vi "Oxford-IPS120-Main.vi"() -> ()   [LabVIEW 2016]
uses:
  IPS120 - SubVIs/Typedefs/Read System 1 - Enum.ctl
  IPS120 - SubVIs/Typedefs/Read System 2 - Enum.ctl
  IPS120 - SubVIs/Typedefs/Read Activity - Enum.ctl
  IPS120 - SubVIs/Typedefs/Read Switch Heater - Enum.ctl
  IPS120 - SubVIs/Typedefs/Read Mode 1 - Enum.ctl
  IPS120 - SubVIs/Typedefs/Read Mode 2 - Enum.ctl
  IPS120 - SubVIs/Typedefs/Set Control - Enum.ctl
  IPS120 - SubVIs/Typedefs/Set Switch Heater - Enum.ctl
  IPS120 - SubVIs/Typedefs/Set Activity - Enum.ctl
  <userlib>/_OpenG.lib/error/error.llb/Filter Error Codes (Array)__ogtk.vi
  API/IPS-120-API.lvlib
  IPS120 - SubVIs/IPS-120.lvlib
panel:
  in  "Tab Control":enum32{"Front Panel", "Error Log"}(tab)=enum."Error Log"
  out "input cluster":T7={"System 1"=enum."Normal", "System 2"=enum."Outside Positive Current Limi", "Activity"=enum."Hold", "Switch Heater"=enum."No Switch Fitted", "Mode 1"=enum."Amps Fast", "Mode 2"=enum."At Rest"}
  out "Magnet Current (A)":dbl=0.0006 format="%.4f"
  out "Voltage (V)":dbl(knob)=-0.0003 scale=-10.0..10.0
  out "Sentinel":bool=TRUE
  in  "Remote Mode":bool
  out "Power Supply Field (T)":dbl=0.0001 format="%#.5f"
  out "Magnet Field (T)":dbl format="%.5f"
  out "Voltage (V)":dbl=-0.0003 format="%.5f"
  out "PS Current (A)":dbl=0.0006 format="%.4f"
  in  "OK":bool
  out "Magnet Field (T)":dbl(knob) caption="Voltage (V)" scale=-20.0..20.0
  out "Switch Time":string="11:11:48"
  in  "PS Heat":bool
  in  "Clamp":bool
  in  "To Set":bool
  in  "To Zero":bool
  in  "Hold":bool
  out "Magnet Status":string="Clamped"
  out "Target Field Rate (T/min)":dbl=1.0 format="%.5f"
  out "Target Field (T)":dbl format="%#.5f"
  in  "Target Rate (T/min)":dbl=0.1 format="%.5f"
  in  "Target Field (T)":dbl format="%#.5f"
  in  "Send to IPS":bool
  out "Current (A)":dbl(knob)=0.0006 scale=-180.0..180.0
  out "Error List":T8(array[cluster])
  in  "IPS120 Address":refnum<visa-resource-name>="GPIB1::24::INSTR"
  # "Current (A)"
  # "Voltage (V)"
  # "Magnet (T)"
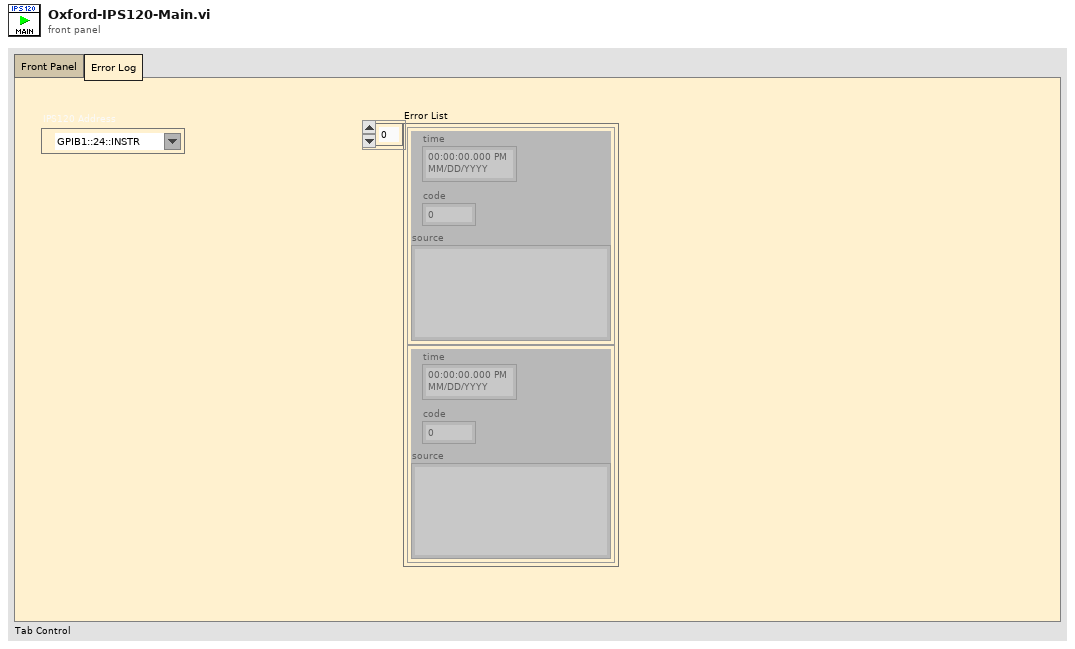
[diagram p1: front panel]
types:
  T1 = typedef "IPS-120.lvlib/Read System 1 - Enum.ctl" = enum16{"Normal", "Quenched", "Over Heated", "Warming Up", "Fault"}
  T2 = typedef "IPS-120.lvlib/Read System 2 - Enum.ctl" = enum16{"Normal", "On Positive Voltage Limit", "On Negative Voltage Limit", "Outside Negative Current Limit", "Outside Positive Current Limi"}
  T3 = typedef "IPS-120.lvlib/Read Activity - Enum.ctl" = enum16{"Hold", "To Set Point", "To Zero", "Clamped"}
  T4 = typedef "IPS-120.lvlib/Read Switch Heater - Enum.ctl" = enum16{"Off Magnet at Zero", "On", "Off Magnet at Field", "Heater Fault", "No Switch Fitted"}
  T5 = typedef "IPS-120.lvlib/Read Mode 1 - Enum.ctl" = enum16{"Amps Fast", "Tesla Fast", "Amps Slow", "Tesla Slow"}
  T6 = typedef "IPS-120.lvlib/Read Mode 2 - Enum.ctl" = enum16{"At Rest", "Sweeping", "Sweep Limiting", "Sweeping & Sweep Limiting"}
  T7 = cluster{"System 1":T1, "System 2":T2, "Activity":T3, "Switch Heater":T4, "Mode 1":T5, "Mode 2":T6}
  T8 = cluster{"time":timestamp, "code":i32, "source":string}[]
  T9 = enum32{"invalid app kind", "Development System", "Run Time System", "Student Edition", "Embedded LabVIEW", "Evaluation", "Custom"}
  T10 = cluster{"time":timestamp, "code":i32, "source":string}
  T11 = enum32{"Invalid", "Standard", "Closed", "Hidden", "Minimized", "Maximized"}
  T12 = typedef "IPS-120.lvlib/Set Control - Enum.ctl" = enum16{"Local & Locked", "Remote & Locked", "Local & Unlocked", "Remote & Unlocked"}
  T13 = cluster{"Magnet Field":dbl, "PS Field":dbl, "Target Field":dbl, "Target Field Rate":dbl, "Voltage":dbl, "Current":dbl, "Switch":bool}
  T14 = cluster{"Target Field (T)":dbl, "Target Field Rate (T/min)":dbl}
  T15 = typedef "IPS-120.lvlib/Set Switch Heater - Enum.ctl" = enum16{"Heater OFF", "Heater ON if PSU=Magnet", "Heater ON, No Checks"}
  T16 = typedef "IPS-120.lvlib/Set Activity - Enum.ctl" = enum16{"Hold", "To Set Point", "To Zero", "Clamp"}
  T17 = cluster{"Core":cluster{"Current VI Reference":refnum<vi>, "Close Panel on Exit?":bool}, "IPS120 Address":refnum<visa-resource-name>, "sentinel":bool, "Error Log":cluster{"time":timestamp, "code":i32, "source":string}[]}
  T18 = typedef "Filtered Error Details - Cluster__ogtk.ctl" = cluster{"code":i32, "source":string}
  T19 = cluster{"Current VI Reference":refnum<vi>, "Close Panel on Exit?":bool}
  T20 = cluster{"System":string, "Activity":string, "Switch Heater":string, "Mode":string}
  T21 = typedef "IPS-120.lvlib/Read X - Cluster.ctl" = cluster{"System 1":T1, "System 2":T2, "Activity":T3, "Switch Heater":T4, "Mode 1":T5, "Mode 2":T6}
  T22 = cluster{"Hold":bool, "Clamp":bool, "To Set":bool, "To Zero":bool, "Send to IPS":bool, "PS Heat":bool}
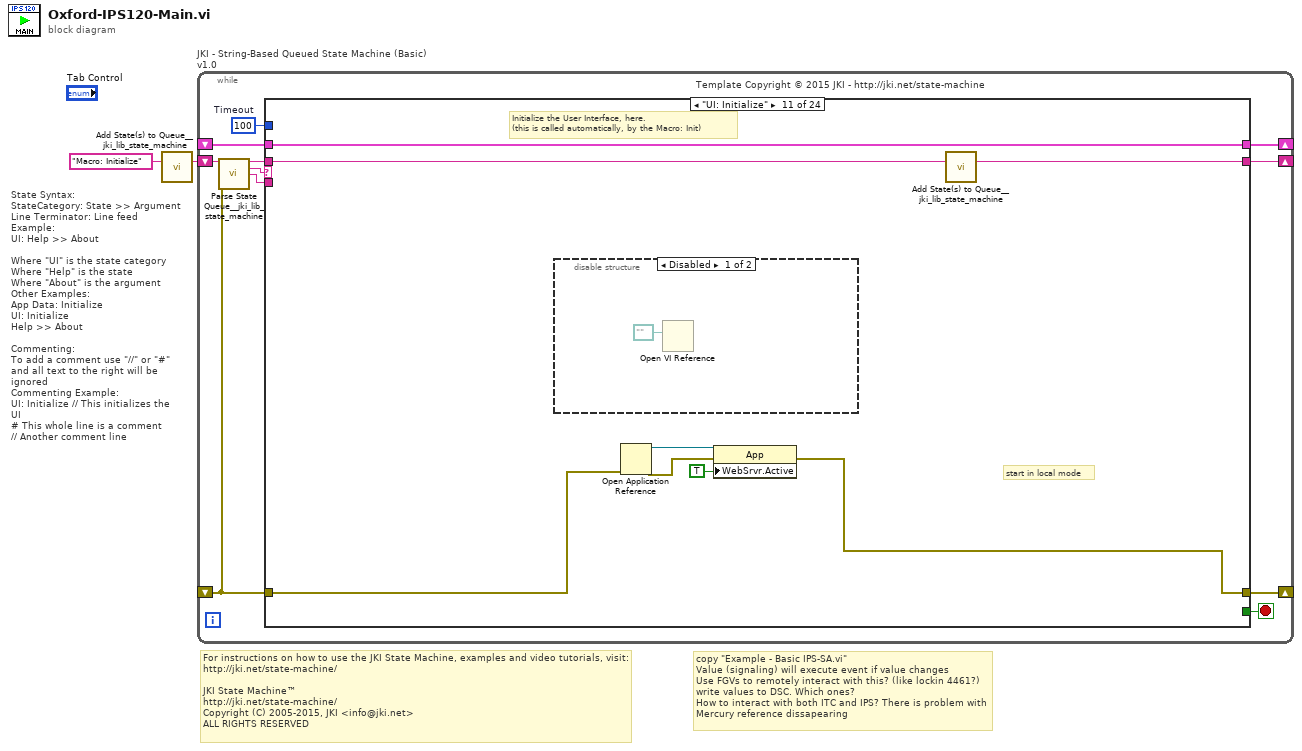
[diagram p0: block diagram]
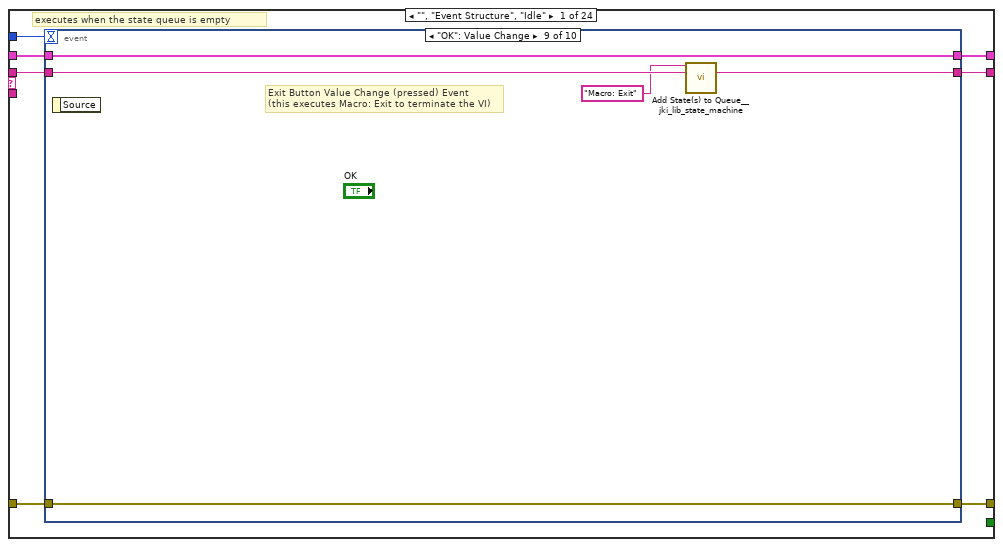
[diagram p2: hidden frame]
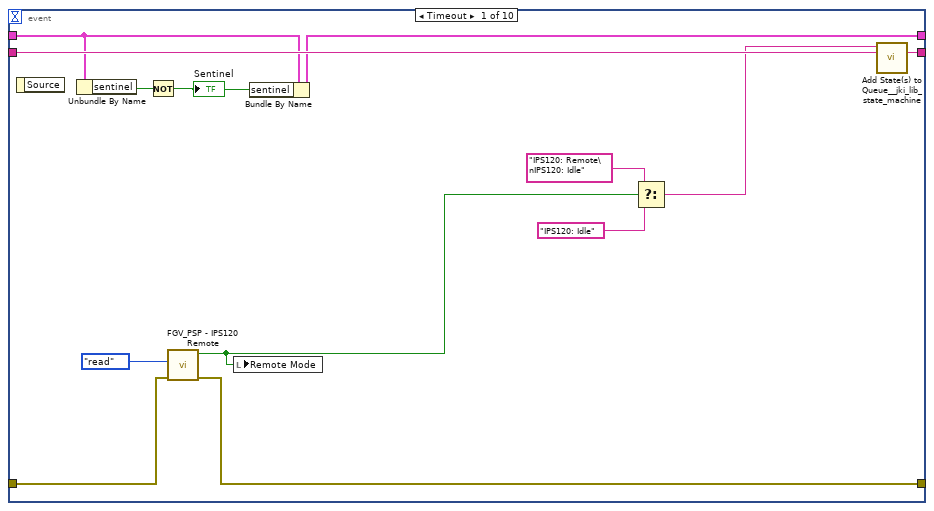
[diagram p3: hidden frame]
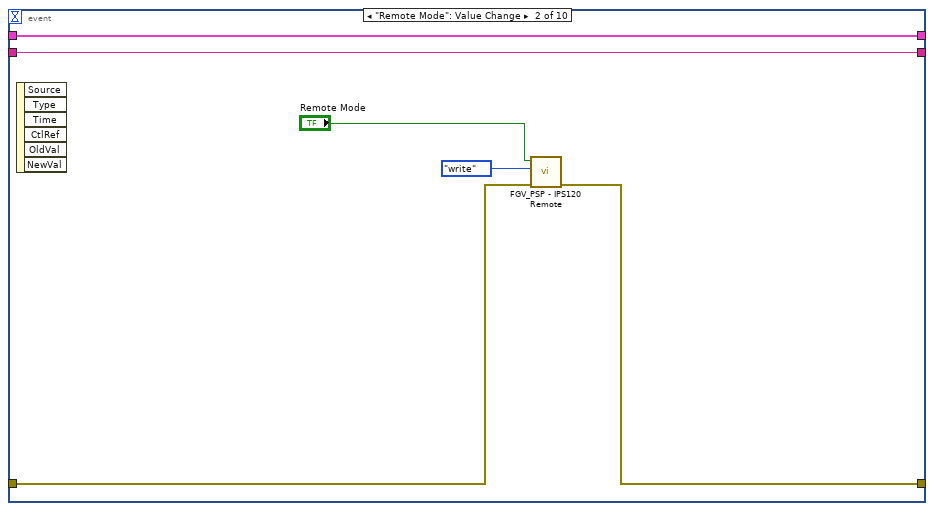
[diagram p4: hidden frame]
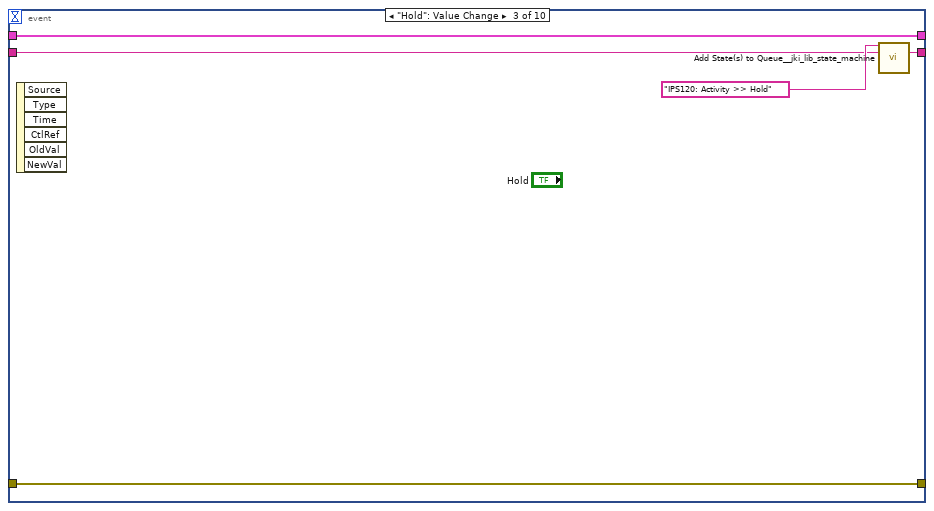
[diagram p5: hidden frame]
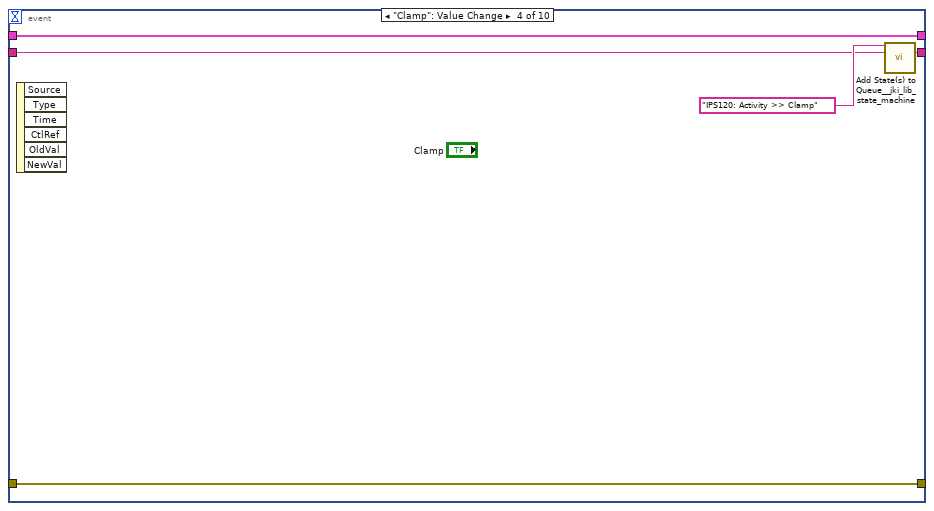
[diagram p6: hidden frame]
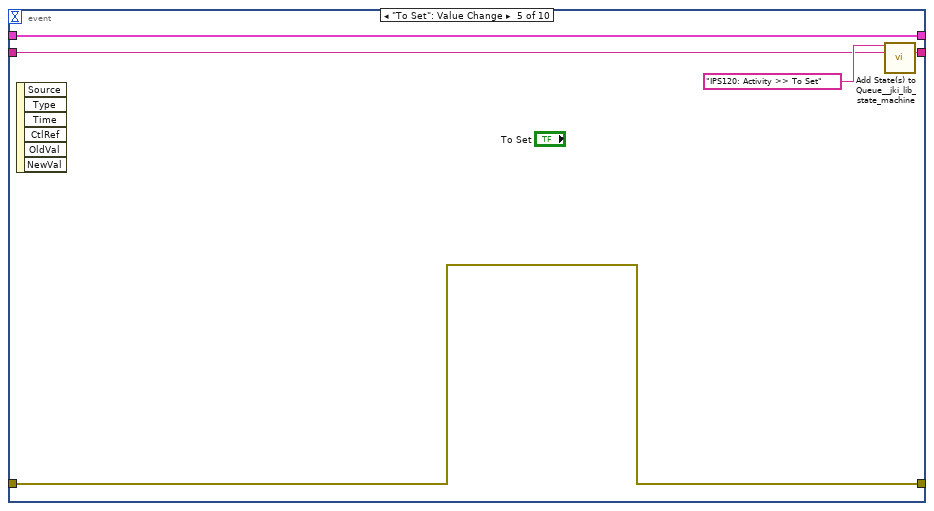
[diagram p7: hidden frame]
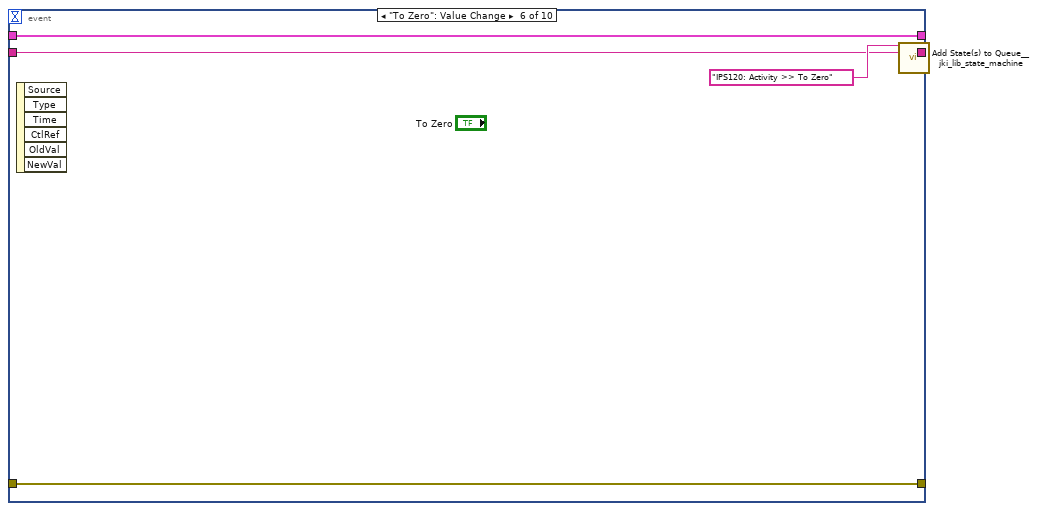
[diagram p8: hidden frame]
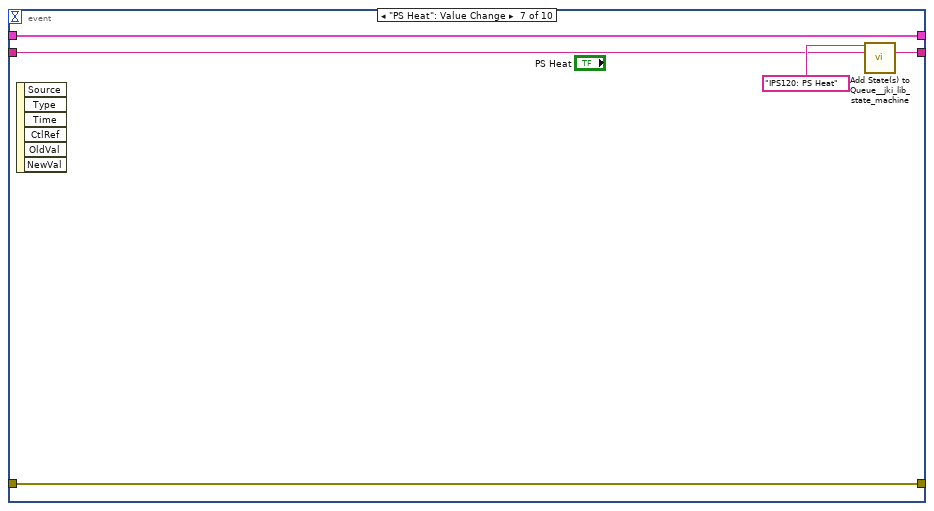
[diagram p9: hidden frame]
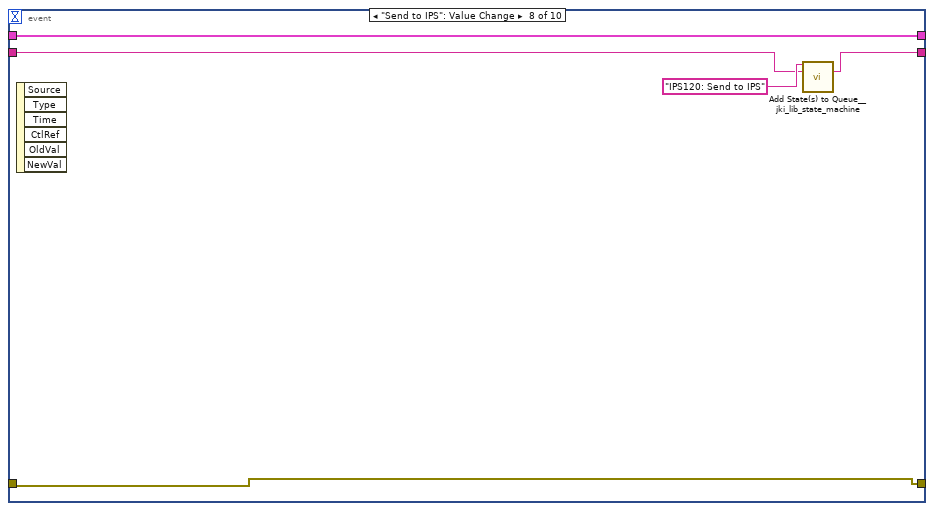
[diagram p10: hidden frame]
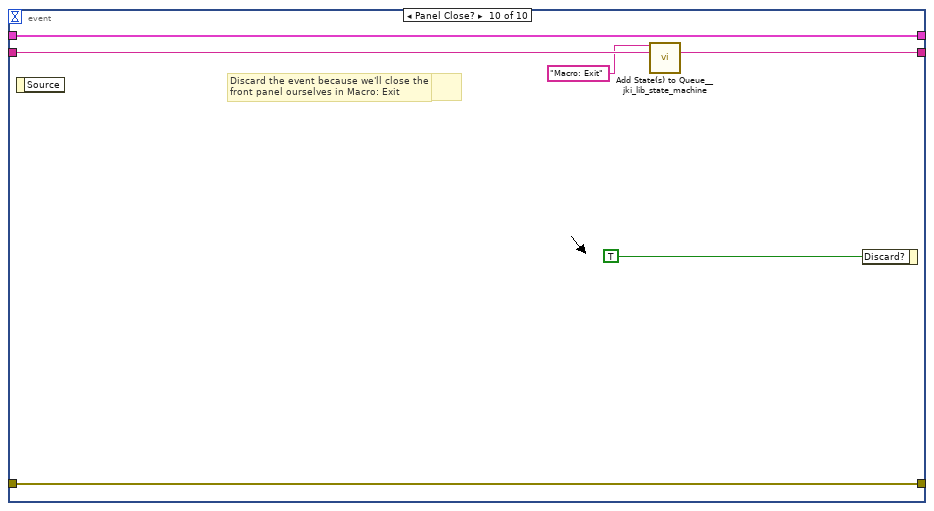
[diagram p11: hidden frame]
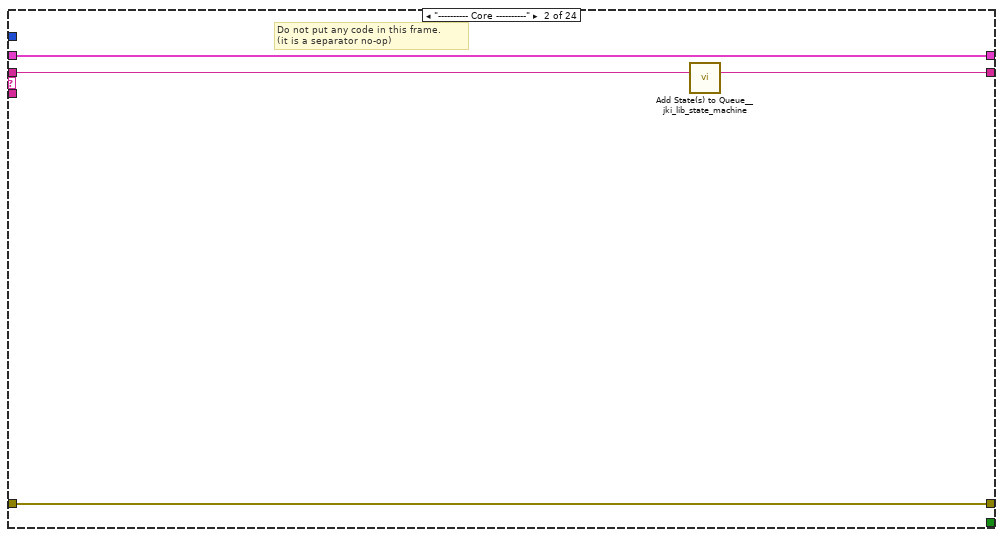
[diagram p12: hidden frame]
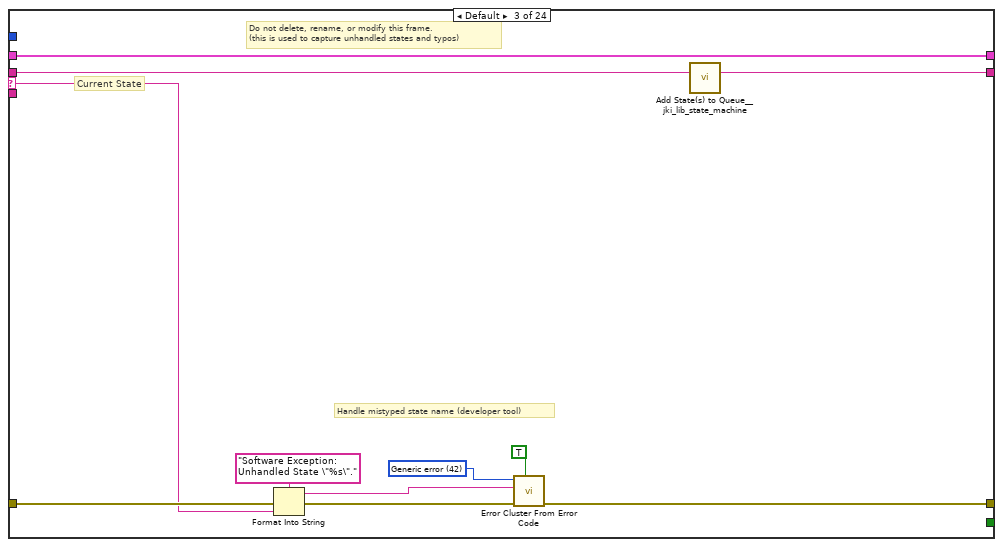
[diagram p13: hidden frame]
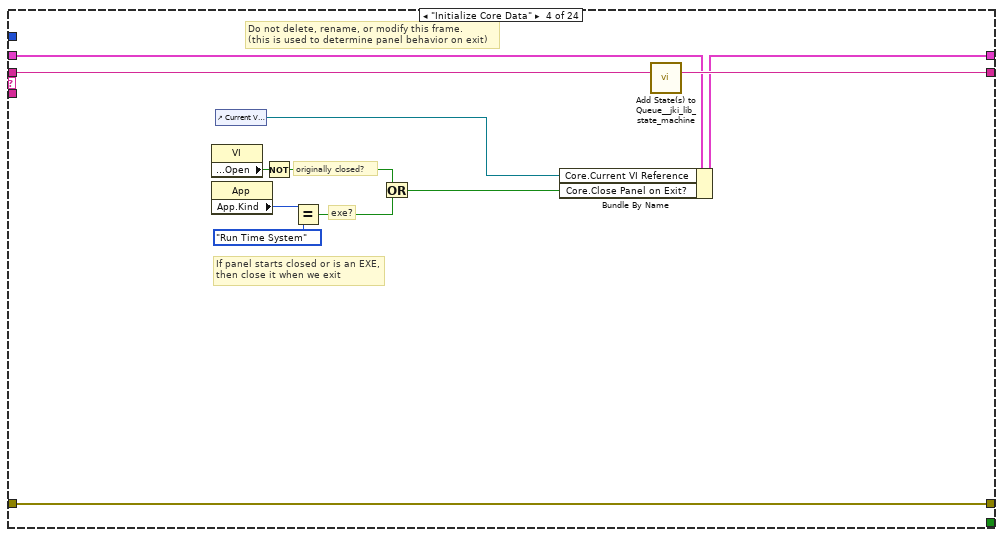
[diagram p14: hidden frame]
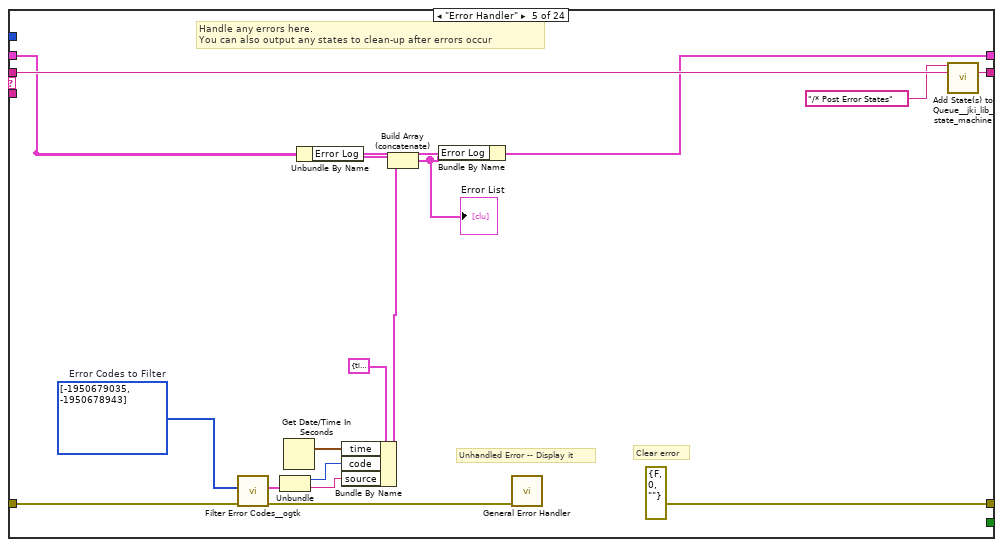
[diagram p15: hidden frame]
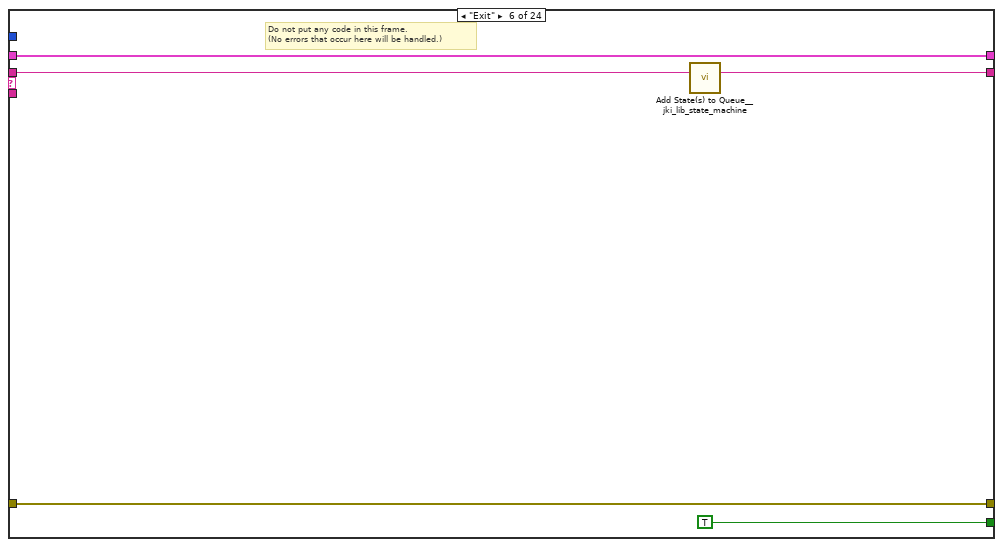
[diagram p16: hidden frame]
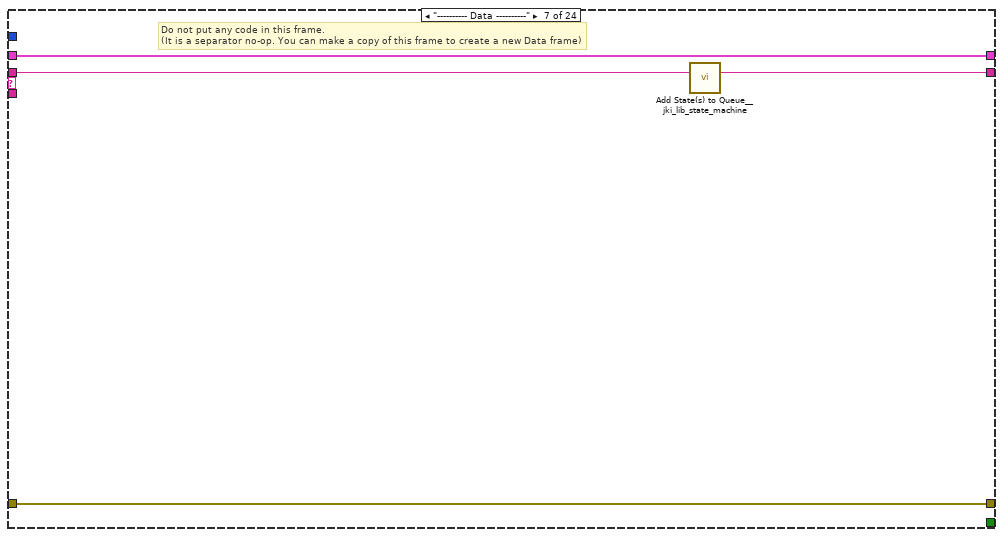
[diagram p17: hidden frame]
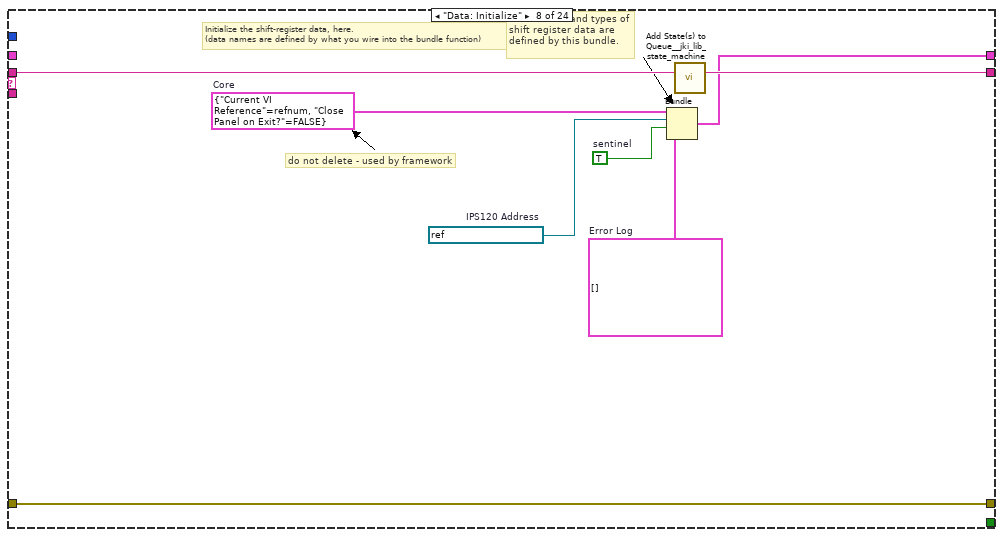
[diagram p18: hidden frame]
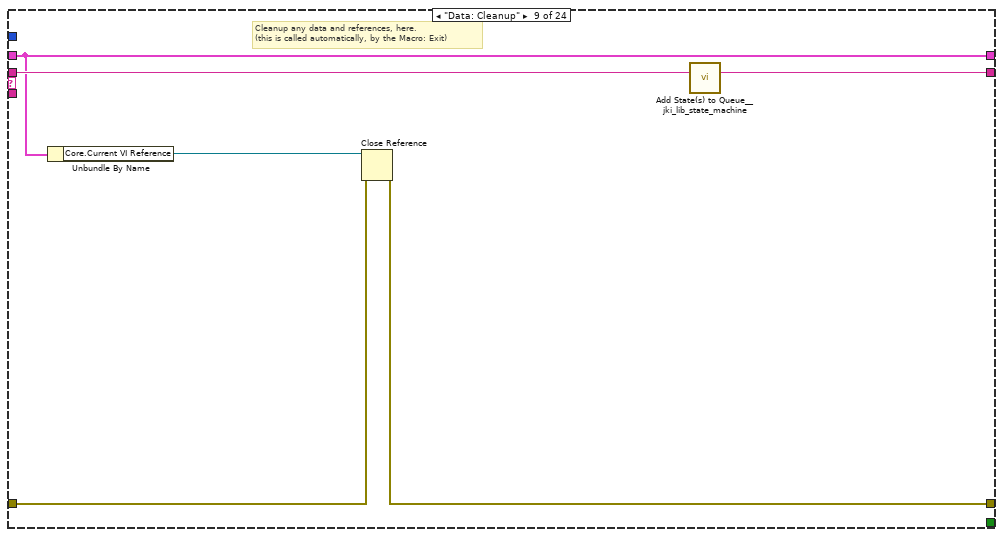
[diagram p19: hidden frame]
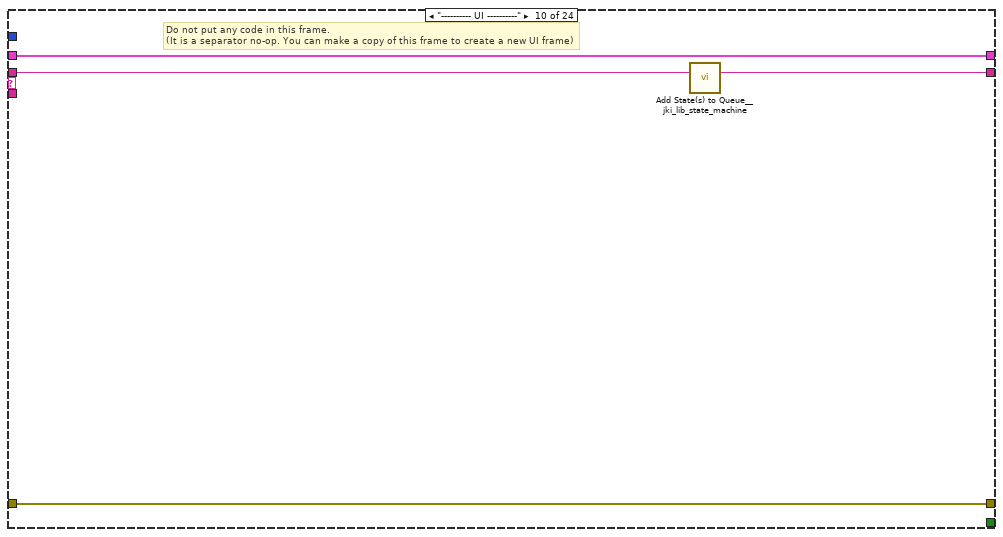
[diagram p20: hidden frame]
diagram:
  # "copy \"Example - Basic IPS-SA.vi\"\nValue (signaling) will execute event if value changes\nUse FGVs to remotely interact with this? (like lockin 4461?)\nwrite values to DSC. Which ones?\nHow to interact with both ITC and IPS? There is problem with \nMercury reference dissapearing"
  # "For instructions on how to use the JKI State Machine, examples and video tutorials, visit:\nhttp://jki.net/state-machine/\n\nJKI State Machine™\nhttp://jki.net/state-machine/\nCopyright (C) 2005-2015, JKI <info@jki.net>\nALL RIGHTS RESERVED"
  # "State Syntax:\nStateCategory: State >> Argument\nLine Terminator: Line feed\nExample:\nUI: Help >> About\n\nWhere \"UI\" is the state category\nWhere \"Help\" is the state\nWhere \"About\" is the argument\nOther Examples:\nApp Data: Initialize\nUI: Initialize\nHelp >> About\n\nCommenting:\nTo add a comment use \"//\" or \"#\" and all text to the right will be ignored\nCommenting Example:\nUI: Initialize // This initializes the UI\n# This whole line is a comment\n// Another comment line"
  n1 = call <vilib>:"Add State(s) to Queue__jki_lib_state_machine.vi"("State(s) in (\"\")"="Macro: Initialize") -> ("States Out"=w2:string)  [unwired: 14 in]
  n2 = while "JKI - String-Based Queued State Machine (Basic) v1.0" {
    shift-right: [w8] -> _
    shift-left: _ -> [w7]
    shift-right: [w11] -> _
    shift-left: _ -> [w5]
    shift-right: [w10] -> _
    shift-left: w2 -> [w12]
    stop <- w9 stop-if-true
    w6 = 100  # Timeout
    # "Template Copyright © 2015 JKI - http://jki.net/state-machine"
    n3 = call <vilib>:"Parse State Queue__jki_lib_state_machine.vi"("State Queue"=w12, "Error In (no error)"=w5) -> ("Remaining States"=w3:string, "Current State"=w4:string, "Arguments"=w13:string)  [unwired: 11 in]
    n4 = case shown="\"UI: Initialize\"" w4 {
      selector: w4 -> [_ _ w85 _ _ _ _ _ _ _ _ _ _ _ _ _ _ _ _ _ _ _ _ _]
      tunnel: w3 -> [w20 w84 w89 w107 w124 w129 w133 w141 w147 w151 w159 w166 w177 w203 w208 w219 w223 w232 w277 w281 w300 w354 w376 w411]
      tunnel: w13 -> [_ _ _ _ _ _ _ _ _ _ _ w161 w171 _ _ _ _ _ _ _ _ _ _ w406]
      tunnel: w7 -> [w16 w81 w87 w98 w110 w127 w130 _ w142 w148 w157 w164 w173 w200 w206 w217 w220 w230 w276 w280 w299 w353 w375 w410]
      tunnel: [w14 w82 w91 w104 errorcluster {"status"=FALSE, "code"=0, "source"=""} ("error out") w126 w131 w136 w143 w149 w152 w162 w174 w201 w205 w210 w221 w225 w234 w279 w292 w346 w364 w405] -> w11
      tunnel: [w19 w83 w88 w106 w123 w128 w132 w140 w146 w150 w158 w165 w176 w202 w207 w218 w222 w231 w278 w282 w301 w355 w377 w412] -> w10
      tunnel: [_ _ _ _ _ TRUE _ _ _ _ _ _ _ _ _ _ _ _ _ _ _ _ _ _] -> w9
      tunnel: [w18 w81 w87 w105 w109 w127 w130 w139 w142 w148 w157 w164 w173 w200 w206 w217 w220 w229 w276 w280 w299 w353 w375 w410] -> w8
      tunnel: w6 -> [w17 _ _ _ _ _ _ _ _ _ _ _ _ _ _ _ _ _ _ _ _ _ _ _]
      tunnel: w5 -> [w15 w82 w90 w104 w119 w126 w131 w136 w144 w149 w153 w163 w175 w201 w205 w209 w221 w226 w265 w279 w296 w347 w365 w407]
      frame "", "Event Structure", "Idle" {
        # "executes when the state queue is empty"
        n5 = event shown="[8] \"OK\": Value Change" {
          selector: _ -> [_ _ _ _ _ _ _ _ _ _]
          dyn-events: _ -> [_ _ _ _ _ _ _ _ _ _]
          timeout: w17 -> [_ _ _ _ _ _ _ _ _ _]
          tunnel: w20 -> [w33 w36 w41 w47 w52 w56 w62 w67 w74 w80]
          tunnel: [w32 w36 w40 w46 w51 w55 w61 w66 w73 w79] -> w19
          tunnel: [w28 w35 w44 w49 w54 w59 w64 w69 w71 w77] -> w18
          tunnel: w16 -> [w29 w35 w44 w49 w54 w59 w64 w69 w71 w77]
          tunnel: w15 -> [w26 w38 w43 w45 w50 w58 w60 w65 w72 w78]
          tunnel: [w25 w37 w43 w45 w50 w58 w60 w65 w72 w78] -> w14
          event Timeout {
            n6 = event-data() -> ()  [unwired: 1 in, 1 out]
            n7 = Unbundle By Name(w29) -> ("sentinel"=w31:bool)
            n8 = Not(x=w31) -> (.not. x?=w30:bool)
            "Sentinel" <- w30
            n9 = call "FGV_PSP - IPS120 Remote.vi"("error in"=w26, "Function"=enum16{"write", "read"}."read") -> ("error out"=w25:errorcluster, "Remote"=w21:bool)  [unwired: 4 in]
            n10 = local write "Remote Mode"(w21) -> ()
            n11 = Bundle By Name(cluster=w29, "sentinel"=w30) -> (w28:T17)
            n12 = Select(t="IPS120: Remote\nIPS120: Idle" ("State(s) in Front (\"\")"), s=w21, f="IPS120: Idle" ("State(s) in Front (\"\")")) -> (s? t:f=w22:string)
            n13 = call <vilib>:"Add State(s) to Queue__jki_lib_state_machine.vi"("State(s) in Front (\"\")"=w22, "State(s) in (\"\")"=w33) -> ("States Out"=w32:string)  [unwired: 13 in]
          }
          event "Remote Mode": Value Change {
            n14 = event-data() -> ()  [unwired: 1 in, 6 out]
            n15 = call "FGV_PSP - IPS120 Remote.vi"("error in"=w38, "Function"=enum16{"write", "read"}."write", "Remote"="Remote Mode") -> ("error out"=w37:errorcluster)  [unwired: 3 in, 1 out]
          }
          event "Hold": Value Change {
            n16 = event-data() -> ()  [unwired: 1 in, 6 out]
            n17 = call <vilib>:"Add State(s) to Queue__jki_lib_state_machine.vi"("State(s) in Front (\"\")"="IPS120: Activity >> Hold" ("State(s) in Front (\"\")"), "State(s) in (\"\")"=w41) -> ("States Out"=w40:string)  [unwired: 13 in]
          }
          event "Clamp": Value Change {
            n18 = event-data() -> ()  [unwired: 1 in, 6 out]
            n19 = call <vilib>:"Add State(s) to Queue__jki_lib_state_machine.vi"("State(s) in Front (\"\")"="IPS120: Activity >> Clamp" ("State(s) in Front (\"\")"), "State(s) in (\"\")"=w47) -> ("States Out"=w46:string)  [unwired: 13 in]
          }
          event "To Set": Value Change {
            n20 = event-data() -> ()  [unwired: 1 in, 6 out]
            n21 = call <vilib>:"Add State(s) to Queue__jki_lib_state_machine.vi"("State(s) in Front (\"\")"="IPS120: Activity >> To Set" ("State(s) in Front (\"\")"), "State(s) in (\"\")"=w52) -> ("States Out"=w51:string)  [unwired: 13 in]
          }
          event "To Zero": Value Change {
            n22 = event-data() -> ()  [unwired: 1 in, 6 out]
            n23 = call <vilib>:"Add State(s) to Queue__jki_lib_state_machine.vi"("State(s) in Front (\"\")"="IPS120: Activity >> To Zero" ("State(s) in Front (\"\")"), "State(s) in (\"\")"=w56) -> ("States Out"=w55:string)  [unwired: 13 in]
          }
          event "PS Heat": Value Change {
            n24 = event-data() -> ()  [unwired: 1 in, 6 out]
            n25 = call <vilib>:"Add State(s) to Queue__jki_lib_state_machine.vi"("State(s) in Front (\"\")"="IPS120: PS Heat", "State(s) in (\"\")"=w62) -> ("States Out"=w61:string)  [unwired: 13 in]
          }
          event "Send to IPS": Value Change {
            n26 = event-data() -> ()  [unwired: 1 in, 6 out]
            n27 = call <vilib>:"Add State(s) to Queue__jki_lib_state_machine.vi"("State(s) in Front (\"\")"="IPS120: Send to IPS", "State(s) in (\"\")"=w67) -> ("States Out"=w66:string)  [unwired: 13 in]
          }
          event "OK": Value Change {
            # "Exit Button Value Change (pressed) Event\n(this executes Macro: Exit to terminate the VI)"
            n28 = event-data() -> ()  [unwired: 1 in, 1 out]
            n29 = call <vilib>:"Add State(s) to Queue__jki_lib_state_machine.vi"("State(s) in Front (\"\")"="Macro: Exit", "State(s) in (\"\")"=w74) -> ("States Out"=w73:string)  [unwired: 13 in]
          }
          event Panel Close? {
            # "Discard the event because we'll close the front panel ourselves in Macro: Exit"
            # "Close Panel button (pressed) Event\n(this executes Macro: Exit to terminate the VI)"
            n30 = event-data() -> ()  [unwired: 1 in, 1 out]
            n31 = call <vilib>:"Add State(s) to Queue__jki_lib_state_machine.vi"("State(s) in Front (\"\")"="Macro: Exit", "State(s) in (\"\")"=w80) -> ("States Out"=w79:string)  [unwired: 13 in]
            n32 = event-data("Discard?"=TRUE) -> ()  [unwired: 1 in, 1 out]
          }
        }
      }
      frame "---------- Core ----------" {
        # "Do not put any code in this frame.\n(it is a separator no-op)"
        n33 = call <vilib>:"Add State(s) to Queue__jki_lib_state_machine.vi"("State(s) in (\"\")"=w84) -> ("States Out"=w83:string)  [unwired: 14 in]
      }
      frame Default {
        w94 = 42 items=["No error", "Argument error", "Memory is full", "Out of zone", "End of file", "File already open", "Generic file I/O error", "File not found", "File permission error", "Disk is full", "Duplicate path", "Too many files open", "System feature not enabled", "Resource file not found", "Cannot add resource", "Resource not found", "Image not found", "Image memory error", "Pen does not exist", "Config type invalid", "Config token not found", "Config parse error", "Config memory error", "Bad external code format", "Bad external code offset", "External code not present", "Null window", "Destroy window error", "Null menu", "Print aborted", "Bad print record", "Print driver error", "Windows error during printing", "Memory error during printing", "Print dialog error", "Generic print error", "Invalid device refnum", "Device not found", "Device parameter error", "Device unit error", "Cannot open device", "Device call aborted", "Generic error", "Cancelled by user", "Object ID too low", "Object ID too high", "Object not in heap", "Unknown heap", "Unknown object (invalid DefProc)", "Unknown object (DefProc not in table)", "Message out of range", "Invalid (null) method", "Unknown message", "Manager call not supported", "Bad address", "Network operation in progress", "Network operation timed out", "Connection is busy", "Network attribute not supported", "Network error", "Address in use", "System out of memory", "Connection aborted", "Connection refused", "Not connected", "Already connected", "Connection closed", "Initialization error (interapplication manager)", "Bad occurrence", "Wait on unbound occurrence handler", "Occurrence queue overflow", "Datalog type conflict", "Unused", "Unrecognized type (interapplication manager)", "Memory corrupt", "Failed to make temporary DLL", "Old CIN version", "Drag socket not found", "Failed to load drop-object", "Failed to register OLE object", "Failed to release OLE object", "Format specifier type mismatch", "Unknown format specifier", "Too few format specifiers", "Too many format specifiers", "Scan failed", "Newer CIN version", "Error converting to variant", "Runtime menu error", "Password tampered", "Variant attribute not found", "Incompatible variant data type", "Event data is not available", "Event Store is not present", "Occurrence is not found", "Event Queue is not created", "Event info is not available", "Refnum passed is NULL", "Error retrieving Class GUID", "Error retrieving CoClass GUID", "Error retrieving TypeLib GUID.", "Bad built application magic bytes.", "Specific driver is different from the specific driver associated with the Logical Name.", "There is no session opened to the class driver.", "Max Error", "MAX - Error with config objects", "MAX - Error loading configuration", "MAX - Group not supported"]
        # "Current State"
        # "Do not delete, rename, or modify this frame.\n(this is used to capture unhandled states and typos)"
        # "Handle mistyped state name (developer tool)"
        n34 = Format Into String(format string="Software Exception: Unhandled State \"%s\"." ("message"), error in=w90, w85) -> (resulting string=w93:string, error out=w92:errorcluster)  [unwired: 1 in]
        n35 = call <vilib>:"Error Cluster From Error Code.vi"("show call chain? (False)"=TRUE, "error in (no error)"=w92, "error message (\"\")"=w93, "error code (0)"=w94) -> ("error out"=w91:errorcluster)  [unwired: 5 in]
        n36 = call <vilib>:"Add State(s) to Queue__jki_lib_state_machine.vi"("State(s) in (\"\")"=w89) -> ("States Out"=w88:string)  [unwired: 14 in]
      }
      frame "Initialize Core Data" {
        # "Do not delete, rename, or modify this frame.\n(this is used to determine panel behavior on exit)"
        # "originally closed?"
        # "exe?"
        # "If panel starts closed or is an EXE, then close it when we exit"
        n37 = property class="VI"() -> ("Front Panel.Open"=w103:bool)  [unwired: 2 in, 2 out]
        n38 = property class="App"() -> ("App.Kind"=w102:T9)  [unwired: 2 in, 2 out]
        n39 = control-ref of="Current VI Reference"() -> (w96:refnum<vi>)
        n40 = Not(x=w103) -> (.not. x?=w100:bool)
        n41 = Equal?(x=w102, y=T9."Run Time System" ("Application:Kind")) -> (x = y?=w99:bool)
        n42 = Or(x=w100, y=w99) -> (x .or. y?=w97:bool)
        n43 = Bundle By Name(cluster=w98, "Core.Current VI Reference"=w96, "Core.Close Panel on Exit?"=w97) -> (w105:T17)
        n44 = call <vilib>:"Add State(s) to Queue__jki_lib_state_machine.vi"("State(s) in (\"\")"=w107) -> ("States Out"=w106:string)  [unwired: 14 in]
      }
      frame "Error Handler" {
        w118 = i32[] [-1950679035, -1950678943]  # Error Codes to Filter
        # "Unhandled Error -- Display it"
        # "Handle any errors here.\nYou can also output any states to clean-up after errors occur"
        # "Clear error"
        n45 = call-poly <userlib>:"Filter Error Codes__ogtk.vi"("Error In"=w119, "Error Codes to Filter"=w118) -> ("Error Out"=w120:errorcluster, "Filtered Error Details"=w117:T18)  [unwired: 7 in, 1 out]
        n46 = Unbundle(w117) -> ("code"=w115:i32, "source"=w116:string)
        n47 = Get Date/Time In Seconds() -> (seconds since 1Jan1904=w114:timestamp)
        n48 = Unbundle By Name(w110) -> ("Error Log"=w112:T8)
        n49 = Bundle By Name(cluster=T10 {"time"=timestamp(0 s since 1904-01-01), "code"=0, "source"=""} ("output cluster"), "time"=w114, "code"=w115, "source"=w116) -> (w111:T10)
        n50 = Build Array (concatenate)(w112, w111) -> (w108:T8)
        "Error List" <- w108
        n51 = Bundle By Name(cluster=w110, "Error Log"=w108) -> (w109:T17)
        n52 = call <vilib>:"General Error Handler.vi"("error in (no error)"=w120) -> ()  [unwired: 10 in, 5 out]
        n53 = call <vilib>:"Add State(s) to Queue__jki_lib_state_machine.vi"("State(s) in Front (\"\")"="/* Post Error States", "State(s) in (\"\")"=w124) -> ("States Out"=w123:string)  [unwired: 13 in]
      }
      frame "Exit" {
        # "Do not put any code in this frame.\n(No errors that occur here will be handled.)"
        n54 = call <vilib>:"Add State(s) to Queue__jki_lib_state_machine.vi"("State(s) in (\"\")"=w129) -> ("States Out"=w128:string)  [unwired: 14 in]
      }
      frame "---------- Data ----------" {
        # "Do not put any code in this frame.\n(It is a separator no-op. You can make a copy of this frame to create a new Data frame)"
        n55 = call <vilib>:"Add State(s) to Queue__jki_lib_state_machine.vi"("State(s) in (\"\")"=w133) -> ("States Out"=w132:string)  [unwired: 14 in]
      }
      frame "Data: Initialize" {
        w134 = refnum<visa-resource-name> "GPIB1::25::INSTR"  # IPS120 Address
        w135 = T8 []  # Error Log
        w137 = TRUE  # sentinel
        w138 = T19 {"Current VI Reference"=refnum, "Close Panel on Exit?"=FALSE}  # Core
        # "do not delete - used by framework"
        # "Data names and types of shift register data are defined by this bundle."
        # "Initialize the shift-register data, here.\n(data names are defined by what you wire into the bundle function)"
        n56 = Bundle("Core"=w138, "IPS120 Address"=w134, "sentinel"=w137, "Error Log"=w135) -> (w139:T17)  [unwired: 1 in]
        n57 = call <vilib>:"Add State(s) to Queue__jki_lib_state_machine.vi"("State(s) in (\"\")"=w141) -> ("States Out"=w140:string)  [unwired: 14 in]
      }
      frame "Data: Cleanup" {
        # "Cleanup any data and references, here.\n(this is called automatically, by the Macro: Exit)"
        n58 = Unbundle By Name(w142) -> ("Core.Current VI Reference"=w145:refnum<vi>)
        n59 = Close Reference(reference=w145, error in (no error)=w144) -> (error out=w143:errorcluster)
        n60 = call <vilib>:"Add State(s) to Queue__jki_lib_state_machine.vi"("State(s) in (\"\")"=w147) -> ("States Out"=w146:string)  [unwired: 14 in]
      }
      frame "---------- UI ----------" {
        # "Do not put any code in this frame.\n(It is a separator no-op. You can make a copy of this frame to create a new UI frame)"
        n61 = call <vilib>:"Add State(s) to Queue__jki_lib_state_machine.vi"("State(s) in (\"\")"=w151) -> ("States Out"=w150:string)  [unwired: 14 in]
      }
      frame "UI: Initialize" {
        # "start in local mode"
        # "Initialize the User Interface, here.\n(this is called automatically, by the Macro: Init)"
        n62 = disable-structure shown="Disabled" {
          frame Disabled {
            n63 = Open VI Reference(vi path=path "") -> ()  [unwired: 5 in, 2 out]
          }
          frame Enabled {
          }
        }
        n64 = Open Application Reference(8:w153) -> (0:w155:errorcluster, 3:w156:refnum<vi>)  [unwired: 3 in]
        n65 = property class="App"(reference=w156, error in=w155, "WebSrvr.Active"=TRUE ("Web Server:Server Active")) -> (error out=w152:errorcluster)  [unwired: 1 out]
        n66 = call <vilib>:"Add State(s) to Queue__jki_lib_state_machine.vi"("State(s) in (\"\")"=w159) -> ("States Out"=w158:string)  [unwired: 14 in]
      }
      frame "UI: Cursor Set" {
        # "Argument"
        # "Set and Unset Cursor Busy.\n(Usage: \"UI: Cursor Set >> Busy|Idle\")"
        n67 = case shown="\"Idle\", Default" w161 {
          tunnel: w163 -> [w168 w170]
          tunnel: [w167 w169] -> w162
          frame "Idle", Default {
            n68 = call <vilib>:"Unset Busy.vi"("error in (no error)"=w168) -> ("error out"=w167:errorcluster)  [unwired: 10 in]
          }
          frame "Busy" {
            n69 = call <vilib>:"Set Busy.vi"("error in (no error)"=w170) -> ("error out"=w169:errorcluster)  [unwired: 9 in, 1 out]
          }
        }
        n70 = call <vilib>:"Add State(s) to Queue__jki_lib_state_machine.vi"("State(s) in (\"\")"=w166) -> ("States Out"=w165:string)  [unwired: 14 in]
      }
      frame "UI: Front Panel State" {
        # "Argument"
        # "Set Front Panel Open or Closed\n(Usage: \"UI: Front Panel State >> Open|Close\")"
        n71 = Unbundle By Name(w173) -> ("Core.Current VI Reference"=w172:refnum<vi>)
        n72 = case shown="\"Open\", Default" w171 {
          tunnel: w175 -> [w181 w194]
          tunnel: [w183 w195] -> w174
          tunnel: w172 -> [w182 w192]
          frame "Open", Default {
            n73 = property class="VI"(reference=w182, error in=w181) -> (reference out=w179:refnum<vi>, error out=w180:errorcluster, "Front Panel.Open"=w178:bool)
            n74 = case shown="True" w178 {
              tunnel: [w186 w189] -> w183
              tunnel: w180 -> [w185 w189]
              tunnel: w179 -> [w184 _]
              frame False {
                n75 = invoke class="VI" method="FP.Open"(reference=w184, error in=w185, "Activate"=TRUE, "State"=T11."Standard") -> (error out=w186:errorcluster)  [unwired: 1 in, 4 out]
              }
              frame True {
              }
            }
          }
          frame "Close" {
            n76 = property class="VI"(reference=w192, error in=w194) -> (reference out=w191:refnum<vi>, error out=w193:errorcluster, "Front Panel.Open"=w190:bool)
            n77 = case shown="True" w190 {
              tunnel: [w196 w199] -> w195
              tunnel: w193 -> [w196 w198]
              tunnel: w191 -> [_ w197]
              frame False {
              }
              frame True {
                n78 = invoke class="VI" method="FP.Close"(reference=w197, error in=w198) -> (error out=w199:errorcluster)  [unwired: 1 in, 2 out]
              }
            }
          }
        }
        n79 = call <vilib>:"Add State(s) to Queue__jki_lib_state_machine.vi"("State(s) in (\"\")"=w177) -> ("States Out"=w176:string)  [unwired: 14 in]
      }
      frame "---------- Macro ----------" {
        # "Do not put any code in this frame.\n(It is a separator no-op. You can make a copy of this frame to create a new Macro frame)"
        n80 = call <vilib>:"Add State(s) to Queue__jki_lib_state_machine.vi"("State(s) in (\"\")"=w203) -> ("States Out"=w202:string)  [unwired: 14 in]
      }
      frame "Macro: Initialize" {
        w204 = "Data: Initialize\nInitialize Core Data\nUI: Initialize\nUI: Front Panel State >> Open\nIPS120: Initialize"  # Data: Initialize Initialize Core Data UI: Initialize UI: Front Panel State >> Open IPS120: Initialize
        # "Initialization Macro\n(This is called once, when the VI starts)"
        n81 = call <vilib>:"Add State(s) to Queue__jki_lib_state_machine.vi"("State(s) in Front (\"\")"=w204, "State(s) in (\"\")"=w208) -> ("States Out"=w207:string)  [unwired: 13 in]
      }
      frame "Macro: Exit" {
        # "Exit Macro\n(This is called once, when the VI exits)"
        n82 = Unbundle By Name(w217) -> ("Core.Close Panel on Exit?"=w216:bool)
        n83 = call <vilib>:"Simple Error Handler.vi"("error in (no error)"=w209) -> ("error out"=w210:errorcluster)  [unwired: 1 in, 7 out]
        n84 = Select(t="UI: Front Panel State >> Close", s=w216, f="") -> (s? t:f=w213:string)
        n85 = call <vilib>:"Add State(s) to Queue__jki_lib_state_machine.vi"("State(s) in (\"\")"=w213, "State(s) at Back (\"\")"="Data: Cleanup\nExit") -> ("States Out"=w211:string)  [unwired: 13 in]
        n86 = call <vilib>:"Add State(s) to Queue__jki_lib_state_machine.vi"("State(s) in Front (\"\")"=w211, "State(s) in (\"\")"=w219) -> ("States Out"=w218:string)  [unwired: 13 in]
      }
      frame "---------- New Category ----------" {
        n87 = call <vilib>:"Add State(s) to Queue__jki_lib_state_machine.vi"("State(s) in (\"\")"=w223) -> ("States Out"=w222:string)  [unwired: 14 in]
      }
      frame "IPS120: Initialize" {
        n88 = call "IPS Set Control.vi"("Error In"=w226, "Control"=Set_Control_-_Enum."Remote & Unlocked", "VISA resource name"="IPS120 Address") -> ("Error Out"=w225:errorcluster, "VISA resource name"=w224:refnum<visa-resource-name>)  [unwired: 2 in, 1 out]
        n89 = Bundle By Name(cluster=w230, "IPS120 Address"=w224) -> (w229:T17)
        n90 = call <vilib>:"Add State(s) to Queue__jki_lib_state_machine.vi"("State(s) in (\"\")"=w232) -> ("States Out"=w231:string)  [unwired: 14 in]
      }
      frame "IPS120: Idle" {
        w236 = enum16{"write", "read"}."write" ("Function")
        n91 = Unbundle By Name(w276) -> ("IPS120 Address"=w264:refnum<visa-resource-name>)
        n92 = call "IPS Read Magnet Field.vi"("Error In"=w265, "VISA resource name"=w264) -> ("Error Out"=w275:errorcluster, "Magnet FIeld (T)"=w246:dbl, "VISA resource name"=w274:refnum<visa-resource-name>)  [unwired: 3 in]
        "Magnet Field (T)" <- w246
        "Magnet Field (T)" <- w246
        n93 = call "IPS Read Target Field.vi"("Error In"=w275, "VISA resource name"=w274) -> ("Error Out"=w273:errorcluster, "Set Point (T)"=w248:dbl, "VISA resource name"=w272:refnum<visa-resource-name>)  [unwired: 3 in]
        "Target Field (T)" <- w248
        n94 = call "IPS Read PS Current.vi"("Error In"=w273, "VISA resource name"=w272) -> ("Error Out"=w271:errorcluster, "Current (A)"=w250:dbl, "VISA resource name"=w270:refnum<visa-resource-name>)  [unwired: 3 in]
        "Current (A)" <- w250
        "PS Current (A)" <- w250
        n95 = call "IPS Read PS Field.vi"("Error In"=w271, "VISA resource name"=w270) -> ("Error Out"=w269:errorcluster, "Field (T)"=w247:dbl, "VISA resource name"=w268:refnum<visa-resource-name>)  [unwired: 3 in]
        "Power Supply Field (T)" <- w247
        n96 = call "IPS Read PS Voltage.vi"("Error In"=w269, "VISA resource name"=w268) -> ("Error Out"=w267:errorcluster, "Power Supply Voltage (V)"=w249:dbl, "VISA resource name"=w266:refnum<visa-resource-name>)  [unwired: 3 in]
        "Voltage (V)" <- w249
        "Voltage (V)" <- w249
        n97 = call "IPS Read Target Field Sweep Rate.vi"("Error In"=w267, "VISA resource name"=w266) -> ("Error Out"=w261:errorcluster, "Field Sweep Rate (T/min)"=w245:dbl, "VISA resource name"=w262:refnum<visa-resource-name>)  [unwired: 3 in]
        "Target Field Rate (T/min)" <- w245
        n98 = call "IPS Read Magnet Current.vi"("Error In"=w261, "VISA resource name"=w262) -> ("Error Out"=w260:errorcluster, "Current (A)"=→"Magnet Current (A)":dbl, "VISA resource name"=w244:refnum<visa-resource-name>)  [unwired: 3 in]
        n99 = Build Array(w246, w248, w250, w247, w245) -> (w238:dbl[])
        n100 = call "IPS Examine Status.vi"("Error In"=w260, "VISA resource name 2"=w244) -> ("Error Out"=w237:errorcluster, "X Strings"=w242:T20, "X Cluster"=w233:T21)  [unwired: 2 in, 1 out]
        "input cluster" <- w233
        n101 = Unbundle By Name(w233) -> ("Switch Heater"=w254:T4, "Activity"=w252:T3, "Mode 2"=w251:T6)
        n102 = Unbundle By Name(w242) -> ("System"=w263:string, "Activity"=w241:string, "Switch Heater"=w240:string, "Mode"=w239:string)
        "Magnet Status" <- w241
        n103 = Equal?(x=Read_Switch_Heater_-_Enum."On" ("Switch Heater"), y=w254) -> (x = y?=w255:bool)
        n104 = Bundle By Name(cluster=T13 {"Magnet Field"=0.0, "PS Field"=0.0, "Target Field"=0.0, "Target Field Rate"=0.0, "Voltage"=0.0, "Current"=0.0, "Switch"=FALSE} ("Status"), "Magnet Field"=w246, "PS Field"=w247, "Target Field"=w248, "Target Field Rate"=w245, "Voltage"=w249, "Current"=w250, "Switch"=w255) -> (w257:T13)
        n105 = call "FGV_PSP - IPS120 Mode Status.vi"("error in"=w237, "Function"=w236, "Mode"=w251) -> ("error out"=w253:errorcluster)  [unwired: 3 in, 1 out]
        n106 = Build Array(w263, w241, w240, w239) -> (w259:string[])
        n107 = call "FGV_PSP - IPS120 Activity Status.vi"("error in"=w253, "Function"=w236, "Activity"=w252) -> ("error out"=w235:errorcluster)  [unwired: 3 in, 1 out]
        n108 = call "IPS120_to_DSC.vi"("str"=w259, "dbl"=w238) -> ()  [unwired: 2 in]
        n109 = call "FGV_PSP - IPS120 Status.vi"("error in"=w235, "Function"=w236, "Status"=w257) -> ("error out"=w234:errorcluster)  [unwired: 3 in, 1 out]
        n110 = call <vilib>:"Add State(s) to Queue__jki_lib_state_machine.vi"("State(s) in (\"\")"=w277) -> ("States Out"=w278:string)  [unwired: 14 in]
      }
      frame "IPS120: Empty" {
        n111 = Unbundle By Name(w280) -> ()  [unwired: 1 out]
        n112 = call <vilib>:"Add State(s) to Queue__jki_lib_state_machine.vi"("State(s) in (\"\")"=w281) -> ("States Out"=w282:string)  [unwired: 14 in]
      }
      frame "IPS120: Send to IPS" {
        w291 = enum16{"write", "read"}."write" ("Function")
        n113 = Unbundle By Name(w299) -> ("IPS120 Address"=w297:refnum<visa-resource-name>)
        n114 = case shown="True" "Send to IPS" {
          tunnel: [w303 w307] -> w286
          tunnel: w297 -> [_ w309]
          tunnel: w296 -> [w303 w308]
          tunnel: [FALSE ("Send to IPS") FALSE ("Send to IPS")] -> w295
          tunnel: [_ "Target Field (T)"] -> w289
          tunnel: [_ "Target Rate (T/min)"] -> w288
          frame False {
          }
          frame True {
            n115 = call "IPS Set Target Field.vi"("Error In"=w308, "Target Field (T)"="Target Field (T)", "VISA resource name"=w309) -> ("Error Out"=w311:errorcluster, "VISA resource name"=w310:refnum<visa-resource-name>)  [unwired: 2 in, 1 out]
            n116 = call "IPS Set Target Field Sweep Rate.vi"("Error In"=w311, "Field Sweep Rate (T/min)"="Target Rate (T/min)", "VISA resource name"=w310) -> ("Error Out"=w307:errorcluster)  [unwired: 2 in, 2 out]
          }
        }
        n117 = local write "Send to IPS"(w295) -> ()
        n118 = call "FGV_PSP - IPS120 Actions.vi"("error in"=w286, "Function"=enum16{"write", "read"}."read") -> ("error out"=w284:errorcluster, "actions"=w283:T22)  [unwired: 4 in]
        n119 = Bundle By Name(cluster=w283, "Send to IPS"=w295) -> (w294:T22)
        n120 = Bundle By Name(cluster=T14 {"Target Field (T)"=0.0, "Target Field Rate (T/min)"=0.0} ("Targets"), "Target Field (T)"=w289, "Target Field Rate (T/min)"=w288) -> (w287:T14)
        n121 = call "FGV_PSP - IPS120 Actions.vi"("error in"=w284, "Function"=w291, "actions"=w294) -> ("error out"=w293:errorcluster)  [unwired: 3 in, 1 out]
        n122 = call "FGV_PSP - IPS120 Targets.vi"("error in"=w293, "Function"=w291, "Targets"=w287) -> ("error out"=w292:errorcluster)  [unwired: 3 in, 1 out]
        n123 = call <vilib>:"Add State(s) to Queue__jki_lib_state_machine.vi"("State(s) in (\"\")"=w300) -> ("States Out"=w301:string)  [unwired: 14 in]
      }
      frame "IPS120: Remote" {
        w330 = "\n"
        w339 = "" ("State(s) in Front (\"\")")
        w351 = enum16{"write", "read"}."read" ("Function")
        n124 = call "FGV_PSP - IPS120 Actions.vi"("error in"=w347, "Function"=w351) -> ("error out"=w352:errorcluster, "actions"=w345:T22)  [unwired: 4 in]
        n125 = Unbundle By Name(w345) -> ("Hold"=w329:bool, "Clamp"=w325:bool, "To Set"=w322:bool, "To Zero"=w313:bool, "Send to IPS"=w312:bool, "PS Heat"=w315:bool)
        n126 = call "FGV_PSP - IPS120 Targets.vi"("error in"=w352, "Function"=w351) -> ("error out"=w346:errorcluster, "Targets"=w350:T14)  [unwired: 4 in]
        n127 = local read "Send to IPS"() -> (w318:bool)
        n128 = Unbundle By Name(w350) -> ("Target Field (T)"=w349:dbl, "Target Field Rate (T/min)"=w348:dbl)
        n129 = local read "To Set"() -> (w323:bool)
        n130 = local read "To Zero"() -> (w320:bool)
        n131 = local read "PS Heat"() -> (w314:bool)
        n132 = local read "Hold"() -> (w328:bool)
        n133 = local read "Clamp"() -> (w326:bool)
        n134 = Not Equal?(x=w328, y=w329) -> (x != y?=w327:bool)
        n135 = Not Equal?(x=w326, y=w325) -> (x != y?=w324:bool)
        n136 = Not Equal?(x=w323, y=w322) -> (x != y?=w321:bool)
        n137 = Not Equal?(x=w320, y=w313) -> (x != y?=w319:bool)
        n138 = Not Equal?(x=w318, y=w312) -> (x != y?=w317:bool)
        n139 = Not Equal?(x=w314, y=w315) -> (x != y?=w316:bool)
        n140 = local write "Hold"(w329) -> ()
        n141 = local write "Clamp"(w325) -> ()
        n142 = local write "To Set"(w322) -> ()
        n143 = local write "To Zero"(w313) -> ()
        n144 = local write "Send to IPS"(w312) -> ()
        n145 = local write "PS Heat"(w315) -> ()
        n146 = local write "Target Field (T)"(w349) -> ()
        n147 = local write "Target Rate (T/min)"(w348) -> ()
        n148 = Select(t="IPS120: Activity >> Hold" ("State(s) in Front (\"\")"), s=w327, f=w339) -> (s? t:f=w336:string)
        n149 = Select(t="IPS120: Activity >> Clamp" ("State(s) in Front (\"\")"), s=w324, f=w339) -> (s? t:f=w335:string)
        n150 = Select(t="IPS120: Activity >> To Set" ("State(s) in Front (\"\")"), s=w321, f=w339) -> (s? t:f=w334:string)
        n151 = Select(t="IPS120: Activity >> To Zero" ("State(s) in Front (\"\")"), s=w319, f=w339) -> (s? t:f=w333:string)
        n152 = Select(t="IPS120: Send to IPS " ("State(s) in Front (\"\")"), s=w317, f=w339) -> (s? t:f=w332:string)
        n153 = Select(t="IPS120: PS Heat" ("State(s) in Front (\"\")"), s=w316, f=w339) -> (s? t:f=w331:string)
        n154 = Concatenate Strings(w336, w330, w335, w330, w334, w330, w333, w330, w332, w330, w331, w330) -> (w340:string)
        n155 = call <vilib>:"Add State(s) to Queue__jki_lib_state_machine.vi"("State(s) in Front (\"\")"=w340, "State(s) in (\"\")"=w354) -> ("States Out"=w355:string)  [unwired: 13 in]
      }
      frame "IPS120: PS Heat" {
        n156 = Unbundle By Name(w375) -> ("IPS120 Address"=w360:refnum<visa-resource-name>)
        n157 = call "IPS Read PS Current.vi"("Error In"=w365, "VISA resource name"=w360) -> ("Error Out"=w369:errorcluster, "Current (A)"=w371:dbl, "VISA resource name"=w368:refnum<visa-resource-name>)  [unwired: 3 in]
        n158 = call "IPS Read Magnet Current.vi"("Error In"=w369, "VISA resource name"=w368) -> ("Error Out"=w367:errorcluster, "Current (A)"=w370:dbl, "VISA resource name"=w366:refnum<visa-resource-name>)  [unwired: 3 in]
        n159 = disable-structure shown="Disabled" {
          disable-tunnel: [w380 TRUE ("T button?")] -> w372
          disable-tunnel: w371 -> [w379 _]
          disable-tunnel: w370 -> [w378 _]
          frame Disabled {
            n160 = Subtract(x=w378, y=w379) -> (x-y=w381:dbl)
            n161 = Absolute Value(x=w381) -> (abs(x)=w382:dbl)
            n162 = Less?(x=w382, y=0.1) -> (x < y?=w384:bool)
            n163 = case shown="False" w384 {
              selector: w384 -> [_ w387]
              tunnel: [w386 w387] -> w380
              frame False {
                n164 = Two Button Dialog(message="The magnet current is more\nthan 0.1A different to the\nPSU output current.  It is not\nadvisable to switch on the\nswitch heater unless these\ncurrents are equal!") -> (T button?=w386:bool)  [unwired: 2 out]
              }
              frame True {
              }
            }
          }
          frame Enabled {
          }
        }
        n165 = local read "PS Heat"() -> (w373:bool)
        n166 = And(x=w373, y=w372) -> (x .and. y?=w374:bool)
        n167 = case shown="True" w374 {
          tunnel: w367 -> [w392 w397]
          tunnel: [w389 w396] -> w363
          tunnel: w366 -> [w391 w398]
          tunnel: [FALSE ("Clamp") TRUE ("Clamp")] -> w359
          frame False {
            n168 = call "IPS Set Switch Heater.vi"("Error In"=w392, "Switch Heater"=Set_Switch_Heater_-_Enum."Heater OFF", "VISA resource name"=w391) -> ("Error Out"=w389:errorcluster)  [unwired: 2 in, 2 out]
          }
          frame True {
            n169 = Get Date/Time In Seconds() -> (seconds since 1Jan1904=w400:timestamp)
            n170 = Get Date/Time String(seconds (now)=w400) -> (time string=→"Switch Time":string)  [unwired: 2 in, 1 out]
            n171 = call "IPS Set Switch Heater.vi"("Error In"=w397, "Switch Heater"=Set_Switch_Heater_-_Enum."Heater ON, No Checks", "VISA resource name"=w398) -> ("Error Out"=w396:errorcluster)  [unwired: 2 in, 2 out]
          }
        }
        n172 = local write "PS Heat"(w359) -> ()
        n173 = call "FGV_PSP - IPS120 Actions.vi"("error in"=w363, "Function"=enum16{"write", "read"}."read") -> ("error out"=w362:errorcluster, "actions"=w358:T22)  [unwired: 4 in]
        n174 = Bundle By Name(cluster=w358, "PS Heat"=w359) -> (w356:T22)
        n175 = call "FGV_PSP - IPS120 Actions.vi"("error in"=w362, "Function"=enum16{"write", "read"}."write", "actions"=w356) -> ("error out"=w364:errorcluster)  [unwired: 3 in, 1 out]
        n176 = call <vilib>:"Add State(s) to Queue__jki_lib_state_machine.vi"("State(s) in (\"\")"=w376) -> ("States Out"=w377:string)  [unwired: 14 in]
      }
      frame "IPS120: Activity" {
        n177 = case shown="\"Hold\", Default" w406 {
          tunnel: [Set_Activity_-_Enum."Hold" ("Set Activity") Set_Activity_-_Enum."To Set Point" ("Set Activity") Set_Activity_-_Enum."To Zero" ("Set Activity") Set_Activity_-_Enum."Clamp" ("Set Activity")] -> w409
          frame "Hold", Default {
          }
          frame "To Set" {
          }
          frame "To Zero" {
          }
          frame "Clamp" {
          }
        }
        n178 = Unbundle By Name(w410) -> ("IPS120 Address"=w408:refnum<visa-resource-name>)
        n179 = call "IPS Set Activity.vi"("Error In"=w407, "Set Activity"=w409, "VISA resource name"=w408) -> ("Error Out"=w403:errorcluster)  [unwired: 2 in, 2 out]
        n180 = call "FGV_PSP - IPS120 Actions.vi"("error in"=w403, "Function"=enum16{"write", "read"}."read") -> ("error out"=w404:errorcluster, "actions"=w401:T22)  [unwired: 4 in]
        n181 = case shown="\"Hold\", Default" w406 {
          tunnel: w404 -> [w416 w422 w428 w433]
          tunnel: [w415 w421 w426 w432] -> w405
          tunnel: w401 -> [w413 w419 w425 w431]
          frame "Hold", Default {
            w414 = FALSE ("Hold")
            n182 = local write "Hold"(w414) -> ()
            n183 = Bundle By Name(cluster=w413, "Hold"=w414) -> (w417:T22)
            n184 = call "FGV_PSP - IPS120 Actions.vi"("error in"=w416, "Function"=enum16{"write", "read"}."write", "actions"=w417) -> ("error out"=w415:errorcluster)  [unwired: 3 in, 1 out]
          }
          frame "To Set" {
            w420 = FALSE ("To Set")
            n185 = local write "To Set"(w420) -> ()
            n186 = Bundle By Name(cluster=w419, "To Set"=w420) -> (w423:T22)
            n187 = call "FGV_PSP - IPS120 Actions.vi"("error in"=w422, "Function"=enum16{"write", "read"}."write", "actions"=w423) -> ("error out"=w421:errorcluster)  [unwired: 3 in, 1 out]
          }
          frame "To Zero" {
            w427 = FALSE ("To Zero")
            n188 = local write "To Zero"(w427) -> ()
            n189 = Bundle By Name(cluster=w425, "To Zero"=w427) -> (w429:T22)
            n190 = call "FGV_PSP - IPS120 Actions.vi"("error in"=w428, "Function"=enum16{"write", "read"}."write", "actions"=w429) -> ("error out"=w426:errorcluster)  [unwired: 3 in, 1 out]
          }
          frame "Clamp" {
            w435 = FALSE ("Clamp")
            n191 = local write "Clamp"(w435) -> ()
            n192 = Bundle By Name(cluster=w431, "Clamp"=w435) -> (w434:T22)
            n193 = call "FGV_PSP - IPS120 Actions.vi"("error in"=w433, "Function"=enum16{"write", "read"}."write", "actions"=w434) -> ("error out"=w432:errorcluster)  [unwired: 3 in, 1 out]
          }
        }
        n194 = call <vilib>:"Add State(s) to Queue__jki_lib_state_machine.vi"("State(s) in (\"\")"=w411) -> ("States Out"=w412:string)  [unwired: 14 in]
      }
    }
  }
